vi "Header-Complete.vi"(8 "error in (no error)":errorcluster) -> (0 "error out":errorcluster, 3 "Headers":string)   [LabVIEW 2013]
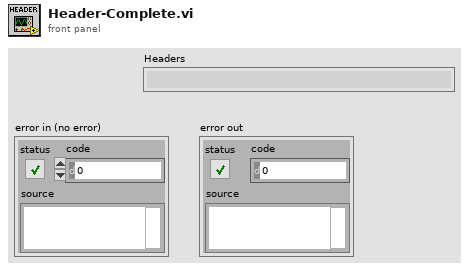
[diagram p1: front panel]
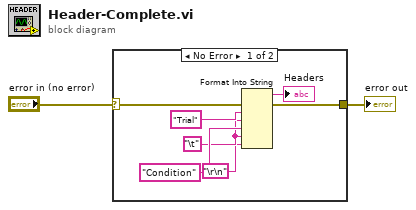
[diagram p0: block diagram]
diagram:
  n1 = case shown="No Error" "error in (no error)" {
    selector: "error in (no error)" -> [w7 w10]
    tunnel: [w8 w10] -> w2
    frame No Error {
      w4 = "\t"
      n2 = Format Into String(error in=w7, "Trial", w4, "Condition" ("format string"), w4, "\r\n") -> (resulting string=→"Headers":string, error out=w8:errorcluster)  [unwired: 2 in]
    }
    frame Error {
    }
  }
  "error out" <- w2
